vi "Estrutura-2.vi"() -> ()   [LabVIEW 2014]
doc: "André Romero - 2016\nandretec@ifsc.usp.br\nIFSC - USP"
panel:
  in  "Zera Motor":bool
  out "stop":bool=TRUE
  out "GetPOS X":dbl format="%#_6f"
  out "GetPOS Y":dbl=-0.00044759115553461015 format="%_6f"
  in  "Graph X":dbl[](array[numeric])=[0.0, 0.0, 0.00044759115553461015, 0.001708984375, 0.0032552082557231188, 0.0052490234375, 0.008097331039607525, 0.011067708022892475, 0.014444987289607525, 0.0189208984375, 0.02315266989171505, 0.02787272073328495, 0.0324300117790699, 0.0380045585334301, 0.0431721992790699, 0.0480550117790699, 0.0526936836540699, 0.0584309883415699, 0.0631103515625, 0.0680338516831398, 0.0735677108168602, 0.0782063826918602, 0.0823567733168602, 0.0860595703125, 0.0898844376206398, 0.0925699844956398, 0.0949300155043602, 0.0968424454331398, 0.0985107421875, 0.0994873046875, 0.099609375, 0.099609375, 0.099609375, 0.099609375, 0.099609375, 0.099609375, 0.099609375, 0.099609375, 0.099609375, 0.099609375, 0.099609375, 0.099609375, 0.099609375, 0.099609375, 0.099609375, 0.099609375, 0.099609375, 0.099609375, 0.099609375, 0.099609375, 0.099609375, 0.099609375, 0.099609375, 0.099609375, 0.099609375, 0.099609375, 0.099609375, 0.099609375, 0.099609375, 0.099609375, 0.1000569686293602, 0.1004231795668602, 0.1015625, 0.1033121719956398, 0.1054280623793602, 0.1078694686293602, 0.1107584610581398, 0.1147867813706398, 0.1185302734375, 0.1228841170668602, 0.1267903596162796, 0.1330973356962204, 0.1380208283662796, 0.1411946564912796, 0.1468912810087204, 0.1532389372587204, 0.1579996794462204, 0.1619466096162796, 0.1681721955537796, 0.173095703125, 0.1763102263212204, 0.1815185546875, 0.1851806640625, 0.1890462189912796, 0.1920166015625, 0.1948649138212204, 0.1964111328125, 0.1982014924287796, 0.19921875, 0.1995442658662796, 0.1995442658662796, 0.1995442658662796, 0.1995442658662796, 0.1995442658662796, 0.1995442658662796, 0.1995442658662796, 0.1995442658662796, 0.1995442658662796, 0.1995442658662796, 0.1995442658662796, 0.1995442658662796, 0.1995442658662796, 0.1995442658662796, 0.1995442658662796, 0.1995442658662796, 0.1995442658662796, 0.1995442658662796, 0.1995442658662796, 0.1995442658662796, 0.1995442658662796, 0.1995442658662796, 0.1995442658662796, 0.1995442658662796, 0.1995442658662796, 0.1995442658662796, 0.1995442658662796, 0.1995442658662796, 0.1995442658662796, 0.1995442658662796, 0.1999918669462204, 0.200439453125, 0.2015787810087204, 0.2030436247587204, 0.2049153596162796, 0.207275390625, 0.2100016325712204, 0.2133382111787796, 0.2169189453125, 0.2209065705537796, 0.22705078125, 0.2318522185087204, 0.23681640625, 0.2414957731962204, 0.2462158203125, 0.2510579526424408, 0.2559000551700592, 0.2623291015625, 0.26708984375, 0.2718505859375, 0.2765706479549408, 0.2809651792049408, 0.2848714292049408, 0.2881673276424408, 0.2921142578125, 0.2946370542049408, 0.2965494692325592, 0.2980550229549408, 0.2991129457950592, 0.2998046875, 0.3000081479549408, 0.3000081479549408, 0.3000081479549408, 0.3000081479549408, 0.3000081479549408, 0.3000081479549408, 0.3000081479549408, 0.3000081479549408, 0.3000081479549408, 0.3000081479549408, 0.3000081479549408, 0.3000081479549408, 0.3000081479549408, 0.3000081479549408, 0.3000081479549408, 0.3000081479549408, 0.3000081479549408, 0.3000081479549408, 0.3000081479549408, 0.3000081479549408, 0.3000081479549408, 0.3000081479549408, 0.3000081479549408, 0.3000081479549408, 0.3000081479549408, 0.3000081479549408, 0.3000081479549408, 0.3000081479549408, 0.3000081479549408, 0.3000081479549408, 0.3000081479549408, 0.3000081479549408, 0.3000081479549408, 0.3000081479549408, 0.3000081479549408, 0.3000081479549408, 0.3000081479549408, 0.3000081479549408, 0.3000081479549408, 0.3000081479549408, 0.3000081479549408, 0.3000081479549408, 0.3000081479549408, 0.3000081479549408, 0.3000081479549408, 0.3000081479549408, 0.3000081479549408, 0.3000081479549408, 0.3000081479549408, 0.2999674379825592, 0.2989501953125, 0.2975260317325592, 0.29541015625, 0.29296875, 0.2903238832950592, 0.2871500551700592, 0.2827962338924408, 0.2786865234375, 0.274169921875, 0.2687174379825592, 0.2638753354549408, 0.2590738832950592, 0.2540283203125, 0.2485758513212204, 0.2436930388212204, 0.2388102263212204, 0.2340901643037796, 0.2284342497587204, 0.2236735075712204, 0.2186279296875, 0.2141520231962204, 0.2085774689912796, 0.2034098356962204, 0.1989339143037796, 0.1941324919462204, 0.1885579377412796, 0.1837565153837204, 0.178955078125, 0.1731363981962204, 0.1686197966337204, 0.1637776643037796, 0.1589762419462204, 0.1533610075712204, 0.1484781950712204, 0.1436767578125, 0.1388753205537796, 0.1332194060087204, 0.1285400390625, 0.1236979141831398, 0.1189778670668602, 0.11328125, 0.1085611954331398, 0.1037190780043602, 0.0980631485581398, 0.09326171875, 0.0884602889418602, 0.0836995467543602, 0.0780843123793602, 0.0732828751206398, 0.068603515625, 0.0636800155043602, 0.0580647774040699, 0.0534261055290699, 0.0483805350959301, 0.043701171875, 0.0380452461540699, 0.0332845039665699, 0.02848307229578495, 0.02376302145421505, 0.01863606832921505, 0.014851887710392475, 0.011433918960392475, 0.007975260727107525, 0.0055745444260537624, 0.0036214191932231188, 0.0017903646221384406, 0.0007731119985692203, 0.00020345051598269492, 0.0, 0.0, -4.069010537932627e-05, -4.069010537932627e-05, 0.0, 0.0, 0.0, 0.0, 0.0, 0.0, 0.0, 0.0, -4.069010537932627e-05, -4.069010537932627e-05, 0.0, 0.0, 0.0, 0.0, 0.0, 0.0, 0.0, 0.0, 0.0, 0.0, 0.0, 0.0, 0.0, 0.0, 0.0]
  in  "Graph Y":dbl[](array[numeric])=[0.0, 0.0, 0.0, 0.0, 0.0, 0.0, 0.0, 0.0, 0.0, 0.0, 0.0, 0.0, 0.0, 0.0, 0.0, 0.0, 0.0, 0.0, 0.0, 0.0, 0.0, 0.0, 0.0, 0.0, 0.0, 0.0, 0.0, 0.0, 0.0, 0.0, 0.0, 0.0, 0.0, 0.0, 0.0, 0.0, 0.0, 0.0, 0.0, 0.0, 0.0, 0.0, 0.0, 0.0, 0.0, 0.0, 0.0, 0.0, 0.0, 0.0, 0.0, 0.0, 0.0, 0.0, 0.0, 0.0, 0.0, 0.0, 0.0, 0.0, 4.069010537932627e-05, 0.0005696614389307797, 0.0017496744403615594, 0.0032552082557231188, 0.0052083334885537624, 0.007568359375, 0.010904948227107525, 0.014200846664607525, 0.01798502542078495, 0.02217610739171505, 0.02689615823328495, 0.0324300117790699, 0.037353515625, 0.0421142578125, 0.0476888008415699, 0.0524088554084301, 0.0572509765625, 0.0620930977165699, 0.067138671875, 0.0716959610581398, 0.0771891251206398, 0.080810546875, 0.0858968123793602, 0.0891520157456398, 0.0916748046875, 0.0948079451918602, 0.0967610701918602, 0.0980224609375, 0.09912109375, 0.099609375, 0.099609375, 0.099609375, 0.099609375, 0.099609375, 0.099609375, 0.099609375, 0.099609375, 0.099609375, 0.099609375, 0.099609375, 0.099609375, 0.099609375, 0.099609375, 0.099609375, 0.099609375, 0.099609375, 0.099609375, 0.099609375, 0.099609375, 0.099609375, 0.099609375, 0.099609375, 0.099609375, 0.099609375, 0.099609375, 0.099609375, 0.099609375, 0.099609375, 0.099609375, 0.1000162735581398, 0.1000162735581398, 0.1000162735581398, 0.1000162735581398, 0.1000162735581398, 0.1000162735581398, 0.1000162735581398, 0.1000162735581398, 0.1000162735581398, 0.1000162735581398, 0.1000162735581398, 0.1000162735581398, 0.1000162735581398, 0.1000162735581398, 0.1000162735581398, 0.1000162735581398, 0.1000162735581398, 0.1000162735581398, 0.1000162735581398, 0.1000162735581398, 0.1000162735581398, 0.1000162735581398, 0.1000162735581398, 0.1000162735581398, 0.1000162735581398, 0.1000162735581398, 0.1000162735581398, 0.1000162735581398, 0.1000162735581398, 0.1000162735581398, 0.0998128280043602, 0.098876953125, 0.09765625, 0.0959065780043602, 0.0937906876206398, 0.0902506485581398, 0.087158203125, 0.0834554061293602, 0.0794270858168602, 0.074951171875, 0.0701090469956398, 0.0653483048081398, 0.0590413399040699, 0.05419921875, 0.04931640625, 0.0445963554084301, 0.0397542305290699, 0.0348714180290699, 0.03019205667078495, 0.02530924417078495, 0.01900227926671505, 0.014200846664607525, 0.009440104477107525, 0.0045979819260537624, -0.000244140625, -0.0064290366135537624, -0.012166340835392475, -0.01611328125, -0.02022298239171505, -0.02657063864171505, -0.03059895895421505, -0.0370279960334301, -0.0417887382209301, -0.0465494804084301, -0.0521647147834301, -0.0569661445915699, -0.061767578125, -0.0666097030043602, -0.0721435546875, -0.076904296875, -0.0811360701918602, -0.0855712890625, -0.0889485701918602, -0.0918782576918602, -0.0942789688706398, -0.0965983048081398, -0.0981038436293602, -0.0992024764418602, -0.0998128280043602, -0.1000162735581398, -0.1000162735581398, -0.1000162735581398, -0.1000162735581398, -0.0999755859375, -0.0999755859375, -0.0999755859375, -0.0999755859375, -0.0999755859375, -0.0999755859375, -0.0999755859375, -0.0999755859375, -0.0999755859375, -0.0999755859375, -0.0999755859375, -0.0999755859375, -0.0999755859375, -0.0999755859375, -0.0999755859375, -0.0999755859375, -0.0999755859375, -0.0999755859375, -0.0999755859375, -0.0999755859375, -0.0999755859375, -0.0999755859375, -0.0999755859375, -0.0999755859375, -0.0999755859375, -0.0999755859375, -0.0999755859375, -0.0999755859375, -0.0999755859375, -0.0999755859375, -0.0999755859375, -0.0999755859375, -0.0999755859375, -0.0999755859375, -0.0999755859375, -0.0999755859375, -0.0999755859375, -0.0999755859375, -0.0999755859375, -0.0999755859375, -0.0999755859375, -0.0999755859375, -0.0999755859375, -0.0999755859375, -0.0999755859375, -0.0999755859375, -0.0999755859375, -0.0999755859375, -0.0999755859375, -0.0999755859375, -0.0999755859375, -0.0999755859375, -0.0999755859375, -0.0999755859375, -0.0999755859375, -0.0999755859375, -0.0999755859375, -0.0999755859375, -0.0999755859375, -0.0999755859375, -0.0999755859375, -0.0999755859375, -0.0999755859375, -0.0999755859375, -0.0999755859375, -0.0994466170668602, -0.0985107421875, -0.0970865860581398, -0.0948893204331398, -0.0925699844956398, -0.0897216796875, -0.0865478515625, -0.0821940079331398, -0.0780029296875, -0.0733642578125, -0.068603515625, -0.0629068985581398, -0.0581461600959301, -0.0533447265625, -0.0478108711540699, -0.04296875, -0.0381266288459301, -0.0333658866584301, -0.02775065042078495, -0.02311197854578495, -0.018798828125, -0.014322916977107525, -0.010945637710392475, -0.008097331039607525, -0.0056559243239462376, -0.0033365886192768812, -0.0018717447528615594, -0.0007731119985692203, -0.00044759115553461015]
  out "XY Graph":cluster{"Graph X":dbl[], "Graph Y":dbl[]}(graph)
  in  "Aceleração":dbl=0.05
  in  "Iniciar":bool
  in  "Velocidade":sgl=0.05
  out "Motor Y\nLigado":bool=TRUE
  out "Motor X \nLigado":bool=TRUE
  # "(mm/s)"
  # "(mm/s.s)"
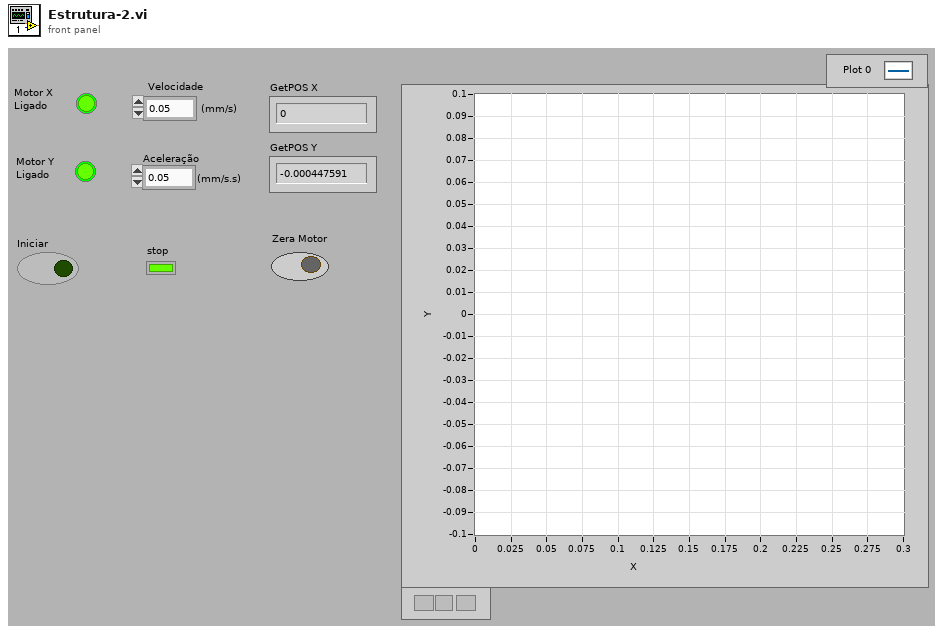
[diagram p1: front panel]
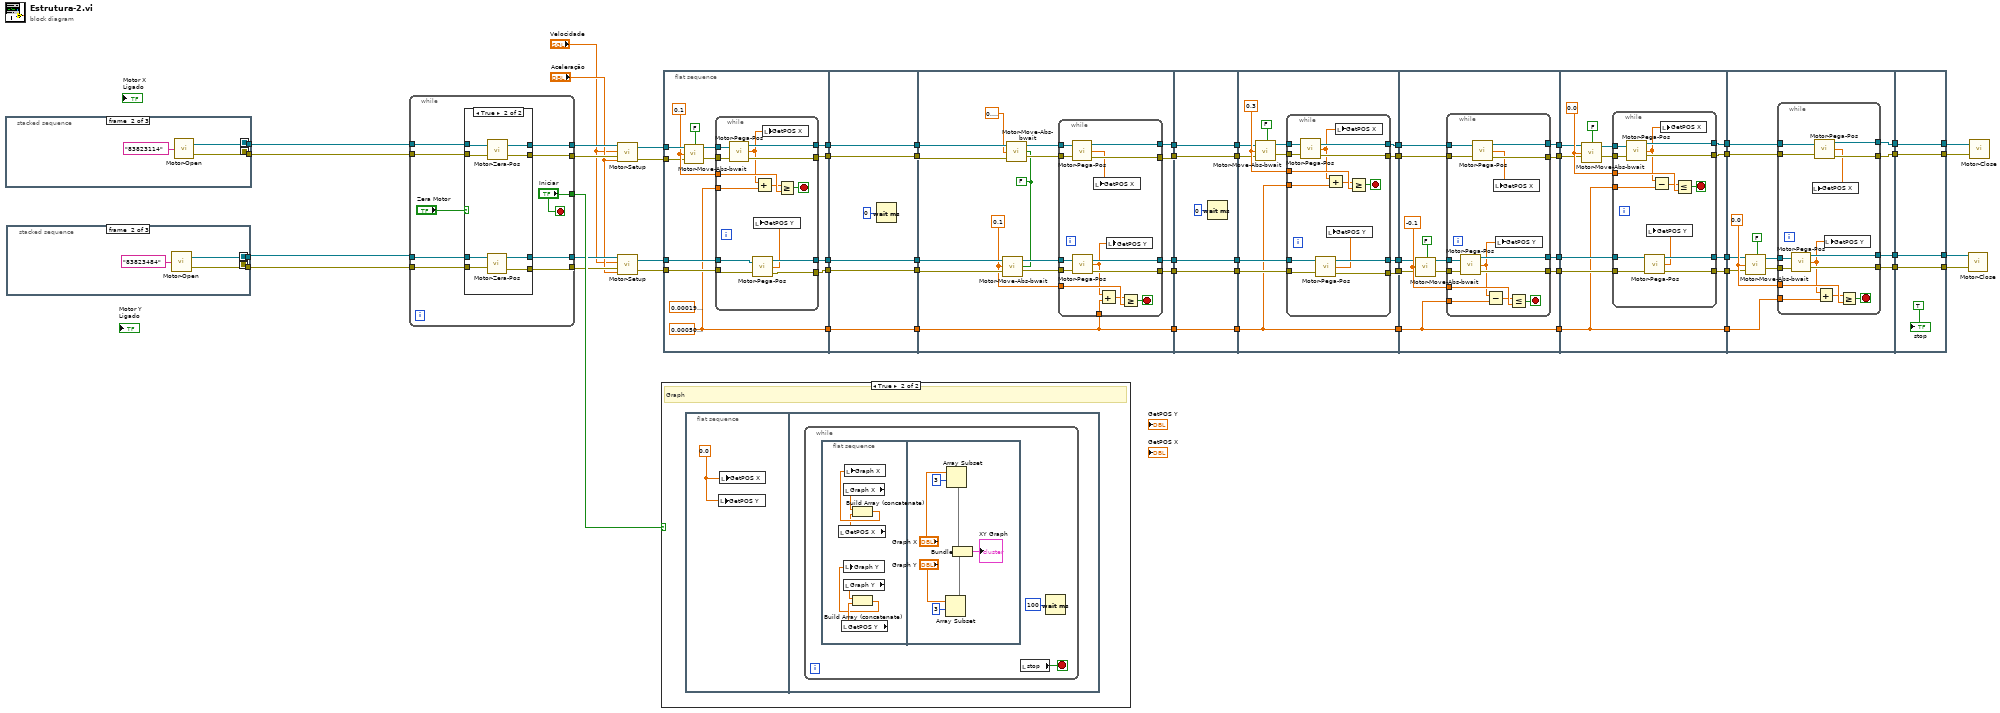
[diagram p0: block diagram]
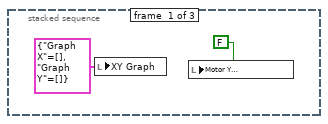
[diagram p4: hidden frame]
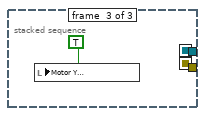
[diagram p5: hidden frame]
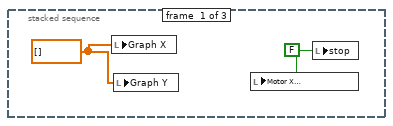
[diagram p6: hidden frame]
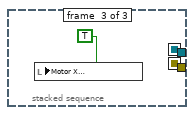
[diagram p7: hidden frame]
diagram:
  n1 = stacked-sequence {
    seq-local: [_ w63 _] -> [_ _ w66]
    seq-local: [_ w62 _] -> [_ _ w65]
    tunnel: [_ _ w66] -> w53
    tunnel: [_ _ w65] -> w52
    frame #0 {
      w59 = dbl[] []
      w60 = FALSE ("x = y?")
      n2 = local write "Graph X"(w59) -> ()
      n3 = local write "Graph Y"(w59) -> ()
      n4 = local write "Motor X \nLigado"(w60) -> ()
      n5 = local write "stop"(w60) -> ()
    }
    frame #1 {
      n6 = call "Motor-Open.vi"("S/N Motor"="83823114") -> ("MG17Motor 2"=w63:refnum<k7>, "error out"=w62:errorcluster)
    }
    frame #2 {
      n7 = local write "Motor X \nLigado"(TRUE ("x = y?")) -> ()
    }
  }
  n8 = stacked-sequence {
    seq-local: [_ w71 _] -> [_ _ w74]
    seq-local: [_ w70 _] -> [_ _ w73]
    tunnel: [_ _ w74] -> w51
    tunnel: [_ _ w73] -> w50
    frame #0 {
      n9 = local write "XY Graph"(cluster{"Graph X":dbl[], "Graph Y":dbl[]} {"Graph X"=[], "Graph Y"=[]} ("XY Graph")) -> ()
      n10 = local write "Motor Y\nLigado"(FALSE ("Motor3\nLigado")) -> ()
    }
    frame #1 {
      n11 = call "Motor-Open.vi"("S/N Motor"="83823484") -> ("MG17Motor 2"=w71:refnum<k7>, "error out"=w70:errorcluster)
    }
    frame #2 {
      n12 = local write "Motor Y\nLigado"(TRUE ("Motor3\nLigado")) -> ()
    }
  }
  n13 = while {
    tunnel: w52 -> [w81]
    tunnel: w50 -> [w79]
    tunnel: [w76] -> w10
    tunnel: [w75] -> w9
    tunnel: [w78] -> w8
    tunnel: [w77] -> w7
    tunnel: w53 -> [w82]
    tunnel: w51 -> [w80]
    tunnel: ["Iniciar"] -> w54
    stop <- "Iniciar" stop-if-true
    n14 = case shown="True" "Zera Motor" {
      tunnel: w82 -> [w88 w96]
      tunnel: w81 -> [w87 w95]
      tunnel: [w88 w94] -> w76
      tunnel: [w87 w93] -> w75
      tunnel: w80 -> [w86 w92]
      tunnel: w79 -> [w85 w91]
      tunnel: [w86 w90] -> w78
      tunnel: [w85 w89] -> w77
      frame False {
      }
      frame True {
        n15 = call "Motor-Zera-Pos.vi"("error"=w91, "MG17Motor A"=w92) -> ("error out"=w89:errorcluster, "MG17Motor out"=w90:refnum<k7>)
        n16 = call "Motor-Zera-Pos.vi"("error"=w95, "MG17Motor A"=w96) -> ("error out"=w93:errorcluster, "MG17Motor out"=w94:refnum<k7>)
      }
    }
  }
  n17 = call "Motor-Setup.vi"("Acc"="Aceleração", "Velocidade"="Velocidade", "error"=w9, "MG17Motor A"=w10) -> ("error out"=w3:errorcluster, "MG17Motor out"=w4:refnum<k7>)
  n18 = call "Motor-Setup.vi"("Acc"="Aceleração", "Velocidade"="Velocidade", "error"=w7, "MG17Motor A"=w8) -> ("error out"=w1:errorcluster, "MG17Motor out"=w2:refnum<k7>)
  n19 = case shown="True" w54 {
    frame False {
    }
    frame True {
      # "Graph"
      n20 = flat-sequence {
        frame #0 {
          w97 = 0.0
          n21 = local write "GetPOS Y"(w97) -> ()
          n22 = local write "GetPOS X"(w97) -> ()
        }
        frame #1 {
          n23 = while {
            stop <- w98 stop-if-true
            n24 = flat-sequence {
              frame #0 {
                n25 = local read "GetPOS X"() -> (w103:dbl)
                n26 = local read "GetPOS Y"() -> (w102:dbl)
                n27 = local read "Graph X"() -> (w105:dbl[])
                n28 = local read "Graph Y"() -> (w100:dbl[])
                n29 = Build Array (concatenate)(w105, w103) -> (w104:dbl[])
                n30 = local write "Graph X"(w104) -> ()
                n31 = Build Array (concatenate)(w100, w102) -> (w101:dbl[])
                n32 = local write "Graph Y"(w101) -> ()
              }
              frame #1 {
                n33 = Array Subset(array="Graph Y", index=3) -> (w106:dbl[])  [unwired: 1 in]
                n34 = Array Subset(array="Graph X", index=3) -> (w109:dbl[])  [unwired: 1 in]
                n35 = Bundle(w109, w106) -> (→"XY Graph":cluster{dbl[], dbl[]})  [unwired: 1 in]
              }
            }
            n36 = local read "stop"() -> (w98:bool)
            n37 = Wait (ms)(milliseconds to wait=u32 100) -> ()  [unwired: 1 out]
          }
        }
      }
    }
  }
  n38 = flat-sequence {
    tunnel: w4 -> [w123]
    tunnel: w3 -> [w121]
    tunnel: [w115] -> w49
    tunnel: w2 -> [w117]
    tunnel: [w114] -> w48
    tunnel: w1 -> [w116]
    tunnel: [w119] -> w47
    tunnel: [w118] -> w46
    tunnel: [w113] -> w45
    tunnel: w49 -> [w145]
    tunnel: [w145] -> w44
    tunnel: w48 -> [w144]
    tunnel: [w144] -> w43
    tunnel: w47 -> [w143]
    tunnel: [w143] -> w42
    tunnel: w46 -> [w142]
    tunnel: [w142] -> w41
    tunnel: w45 -> [w141]
    tunnel: [w141] -> w40
    tunnel: w44 -> [w159]
    tunnel: w43 -> [w158]
    tunnel: [w155] -> w39
    tunnel: w42 -> [w152]
    tunnel: w41 -> [w149]
    tunnel: [w154] -> w38
    tunnel: [w157] -> w37
    tunnel: [w156] -> w36
    tunnel: w40 -> [w153]
    tunnel: [w153] -> w35
    tunnel: w39 -> [w181]
    tunnel: [w181] -> w34
    tunnel: w38 -> [w180]
    tunnel: [w180] -> w33
    tunnel: w37 -> [w179]
    tunnel: [w179] -> w32
    tunnel: w36 -> [w178]
    tunnel: [w178] -> w31
    tunnel: w35 -> [w177]
    tunnel: [w177] -> w30
    tunnel: w34 -> [w190]
    tunnel: w33 -> [w189]
    tunnel: w32 -> [w185]
    tunnel: [w183] -> w29
    tunnel: w31 -> [w186]
    tunnel: [w184] -> w28
    tunnel: [w188] -> w27
    tunnel: [w187] -> w26
    tunnel: w30 -> [w182]
    tunnel: [w182] -> w25
    tunnel: w29 -> [w216]
    tunnel: w28 -> [w217]
    tunnel: w27 -> [w213]
    tunnel: [w211] -> w24
    tunnel: w26 -> [w212]
    tunnel: [w210] -> w23
    tunnel: [w215] -> w22
    tunnel: [w214] -> w21
    tunnel: w25 -> [w209]
    tunnel: [w209] -> w20
    tunnel: w24 -> [w243]
    tunnel: w23 -> [w244]
    tunnel: w22 -> [w240]
    tunnel: w21 -> [w239]
    tunnel: [w242] -> w19
    tunnel: [w241] -> w18
    tunnel: [w238] -> w17
    tunnel: [w237] -> w16
    tunnel: w20 -> [w236]
    tunnel: [w236] -> w15
    tunnel: w19 -> [w267]
    tunnel: w18 -> [w266]
    tunnel: w17 -> [w271]
    tunnel: w16 -> [w270]
    tunnel: [w265] -> w14
    tunnel: [w264] -> w13
    tunnel: [w269] -> w12
    tunnel: [w268] -> w11
    tunnel: w15 -> [w263]
    tunnel: [w291] -> w55
    tunnel: [w292] -> w56
    tunnel: [w293] -> w57
    tunnel: [w294] -> w58
    tunnel: w14 -> [w294]
    tunnel: w13 -> [w293]
    tunnel: w12 -> [w292]
    tunnel: w11 -> [w291]
    frame #0 {
      (unwired) sgl 0.0002 ("y")
      w113 = sgl 0.0005 ("y")
      w122 = 0.1
      n39 = call "Motor-Move-Abs-bwait.vi"("bWait"=FALSE, "error"=w121, "Posição"=w122, "MG17Motor A"=w123) -> ("error out"=w124:errorcluster, "MG17Motor out"=w125:refnum<k7>)
      n40 = while {
        tunnel: w125 -> [w139]
        tunnel: w124 -> [w138]
        tunnel: w122 -> [w136]
        tunnel: [w134] -> w119
        tunnel: [w133] -> w118
        tunnel: w117 -> [w131]
        tunnel: w116 -> [w130]
        tunnel: [w129] -> w115
        tunnel: [w128] -> w114
        tunnel: w113 -> [w126]
        stop <- w137 stop-if-true
        n41 = call "Motor-Pega-Pos.vi"("MG17Motor 2"=w139, "error out"=w138) -> ("MG17Motor 3"=w134:refnum<k7>, "pfPosition"=w132:sgl, "error out 2"=w133:errorcluster)
        n42 = call "Motor-Pega-Pos.vi"("MG17Motor 2"=w131, "error out"=w130) -> ("MG17Motor 3"=w129:refnum<k7>, "pfPosition"=w127:sgl, "error out 2"=w128:errorcluster)
        n43 = local write "GetPOS Y"(w127) -> ()
        n44 = Add(x=w132, y=w126) -> (x+y=w135:sgl)
        n45 = local write "GetPOS X"(w132) -> ()
        n46 = Greater Or Equal?(x=w135, y=w136) -> (x >= y?=w137:bool)
      }
    }
    frame #1 {
      n47 = Wait (ms)(milliseconds to wait=u32 0) -> ()  [unwired: 1 out]
    }
    frame #2 {
      w147 = FALSE
      w148 = 0.1
      n48 = call "Motor-Move-Abs-bwait.vi"("bWait"=w147, "error"=w158, "Posição"=w148, "MG17Motor A"=w159) -> ("error out"=w160:errorcluster, "MG17Motor out"=w161:refnum<k7>)
      n49 = call "Motor-Move-Abs-bwait.vi"("bWait"=w147, "error"=w149, "Posição"=sgl 0.2, "MG17Motor A"=w152) -> ("error out"=w150:errorcluster, "MG17Motor out"=w151:refnum<k7>)
      n50 = while {
        tunnel: w161 -> [w175]
        tunnel: w160 -> [w174]
        tunnel: w148 -> [w172]
        tunnel: [w170] -> w157
        tunnel: [w169] -> w156
        tunnel: w151 -> [w167]
        tunnel: w150 -> [w166]
        tunnel: [w165] -> w155
        tunnel: [w164] -> w154
        tunnel: w153 -> [w162]
        stop <- w173 stop-if-true
        n51 = call "Motor-Pega-Pos.vi"("MG17Motor 2"=w167, "error out"=w166) -> ("MG17Motor 3"=w165:refnum<k7>, "pfPosition"=w163:sgl, "error out 2"=w164:errorcluster)
        n52 = call "Motor-Pega-Pos.vi"("MG17Motor 2"=w175, "error out"=w174) -> ("MG17Motor 3"=w169:refnum<k7>, "pfPosition"=w168:sgl, "error out 2"=w170:errorcluster)
        n53 = local write "GetPOS X"(w163) -> ()
        n54 = Add(x=w168, y=w162) -> (x+y=w171:sgl)
        n55 = local write "GetPOS Y"(w168) -> ()
        n56 = Greater Or Equal?(x=w171, y=w172) -> (x >= y?=w173:bool)
      }
    }
    frame #3 {
      n57 = Wait (ms)(milliseconds to wait=u32 0) -> ()  [unwired: 1 out]
    }
    frame #4 {
      w192 = 0.3
      n58 = call "Motor-Move-Abs-bwait.vi"("bWait"=FALSE, "error"=w189, "Posição"=w192, "MG17Motor A"=w190) -> ("error out"=w193:errorcluster, "MG17Motor out"=w194:refnum<k7>)
      n59 = while {
        tunnel: w194 -> [w208]
        tunnel: w193 -> [w207]
        tunnel: w192 -> [w205]
        tunnel: [w203] -> w188
        tunnel: [w202] -> w187
        tunnel: w186 -> [w200]
        tunnel: w185 -> [w199]
        tunnel: [w198] -> w184
        tunnel: [w197] -> w183
        tunnel: w182 -> [w195]
        stop <- w206 stop-if-true
        n60 = call "Motor-Pega-Pos.vi"("MG17Motor 2"=w208, "error out"=w207) -> ("MG17Motor 3"=w203:refnum<k7>, "pfPosition"=w201:sgl, "error out 2"=w202:errorcluster)
        n61 = call "Motor-Pega-Pos.vi"("MG17Motor 2"=w200, "error out"=w199) -> ("MG17Motor 3"=w198:refnum<k7>, "pfPosition"=w196:sgl, "error out 2"=w197:errorcluster)
        n62 = Add(x=w201, y=w195) -> (x+y=w204:sgl)
        n63 = local write "GetPOS Y"(w196) -> ()
        n64 = local write "GetPOS X"(w201) -> ()
        n65 = Greater Or Equal?(x=w204, y=w205) -> (x >= y?=w206:bool)
      }
    }
    frame #5 {
      w219 = -0.1
      n66 = call "Motor-Move-Abs-bwait.vi"("bWait"=FALSE, "error"=w216, "Posição"=w219, "MG17Motor A"=w217) -> ("error out"=w220:errorcluster, "MG17Motor out"=w221:refnum<k7>)
      n67 = while {
        tunnel: w221 -> [w235]
        tunnel: w220 -> [w234]
        tunnel: w219 -> [w232]
        tunnel: [w230] -> w215
        tunnel: [w229] -> w214
        tunnel: w213 -> [w227]
        tunnel: w212 -> [w226]
        tunnel: [w225] -> w211
        tunnel: [w224] -> w210
        tunnel: w209 -> [w222]
        stop <- w233 stop-if-true
        n68 = call "Motor-Pega-Pos.vi"("MG17Motor 2"=w235, "error out"=w234) -> ("MG17Motor 3"=w230:refnum<k7>, "pfPosition"=w228:sgl, "error out 2"=w229:errorcluster)
        n69 = call "Motor-Pega-Pos.vi"("MG17Motor 2"=w227, "error out"=w226) -> ("MG17Motor 3"=w225:refnum<k7>, "pfPosition"=w223:sgl, "error out 2"=w224:errorcluster)
        n70 = Subtract(x=w228, y=w222) -> (x-y=w231:sgl)
        n71 = local write "GetPOS X"(w223) -> ()
        n72 = local write "GetPOS Y"(w228) -> ()
        n73 = Less Or Equal?(x=w231, y=w232) -> (x <= y?=w233:bool)
      }
    }
    frame #6 {
      w246 = 0.0
      n74 = call "Motor-Move-Abs-bwait.vi"("bWait"=FALSE, "error"=w244, "Posição"=w246, "MG17Motor A"=w243) -> ("error out"=w247:errorcluster, "MG17Motor out"=w248:refnum<k7>)
      n75 = while {
        tunnel: w248 -> [w262]
        tunnel: w247 -> [w261]
        tunnel: w246 -> [w259]
        tunnel: [w257] -> w242
        tunnel: [w256] -> w241
        tunnel: w240 -> [w254]
        tunnel: w239 -> [w253]
        tunnel: [w252] -> w238
        tunnel: [w251] -> w237
        tunnel: w236 -> [w249]
        stop <- w260 stop-if-true
        n76 = call "Motor-Pega-Pos.vi"("MG17Motor 2"=w262, "error out"=w261) -> ("MG17Motor 3"=w257:refnum<k7>, "pfPosition"=w255:sgl, "error out 2"=w256:errorcluster)
        n77 = call "Motor-Pega-Pos.vi"("MG17Motor 2"=w254, "error out"=w253) -> ("MG17Motor 3"=w252:refnum<k7>, "pfPosition"=w250:sgl, "error out 2"=w251:errorcluster)
        n78 = local write "GetPOS Y"(w250) -> ()
        n79 = Subtract(x=w255, y=w249) -> (x-y=w258:sgl)
        n80 = local write "GetPOS X"(w255) -> ()
        n81 = Less Or Equal?(x=w258, y=w259) -> (x <= y?=w260:bool)
      }
    }
    frame #7 {
      w274 = 0.0
      n82 = call "Motor-Move-Abs-bwait.vi"("bWait"=FALSE, "error"=w270, "Posição"=w274, "MG17Motor A"=w271) -> ("error out"=w273:errorcluster, "MG17Motor out"=w272:refnum<k7>)
      n83 = while {
        tunnel: w272 -> [w289]
        tunnel: w273 -> [w288]
        tunnel: w274 -> [w286]
        tunnel: [w284] -> w269
        tunnel: [w283] -> w268
        tunnel: w267 -> [w281]
        tunnel: w266 -> [w280]
        tunnel: [w279] -> w265
        tunnel: [w278] -> w264
        tunnel: w263 -> [w276]
        stop <- w287 stop-if-true
        n84 = call "Motor-Pega-Pos.vi"("MG17Motor 2"=w289, "error out"=w288) -> ("MG17Motor 3"=w284:refnum<k7>, "pfPosition"=w282:sgl, "error out 2"=w283:errorcluster)
        n85 = call "Motor-Pega-Pos.vi"("MG17Motor 2"=w281, "error out"=w280) -> ("MG17Motor 3"=w279:refnum<k7>, "pfPosition"=w277:sgl, "error out 2"=w278:errorcluster)
        n86 = local write "GetPOS X"(w277) -> ()
        n87 = Add(x=w282, y=w276) -> (x+y=w285:sgl)
        n88 = local write "GetPOS Y"(w282) -> ()
        n89 = Greater Or Equal?(x=w285, y=w286) -> (x >= y?=w287:bool)
      }
    }
    frame #8 {
      "stop" <- TRUE ("stop")
    }
  }
  n90 = call "Motor-Close.vi"("error out"=w55, "MG17Motor 3"=w56) -> ()  [unwired: 1 in]
  n91 = call "Motor-Close.vi"("error out"=w57, "MG17Motor 3"=w58) -> ()  [unwired: 1 in]
